vi "SkipIfLabVIEWVersionIsIncompatible.vi"(8 "error in (no error)":errorcluster, 10 "Minimum Version Year (2016)":string="2016", 11 "VeriStandTestCase in":refnum<class "VeriStandTestCase.lvclass">) -> (0 "error out":errorcluster, 2 "Skipped":bool, 3 "VeriStandTestCase out":refnum<class "VeriStandTestCase.lvclass">)   [LabVIEW 2027, in "VeriStandTestCase.lvclass"]
uses:
  VeriStandTestCase.lvclass
  <vilib>/addons/_JKI Toolkits/VI Tester/TestCase.llb/TestCase.lvclass
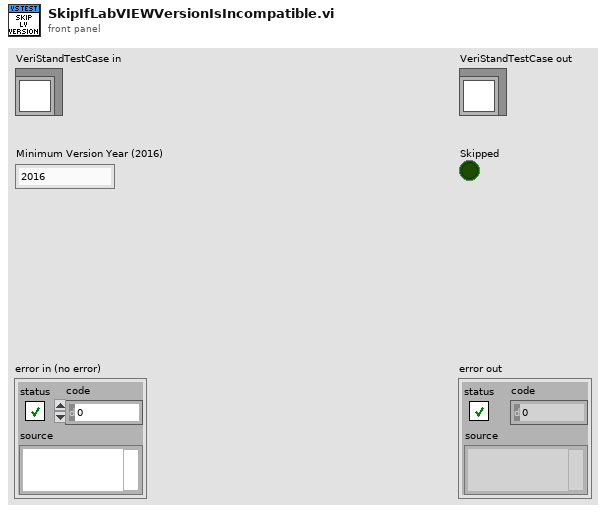
[diagram p1: front panel]
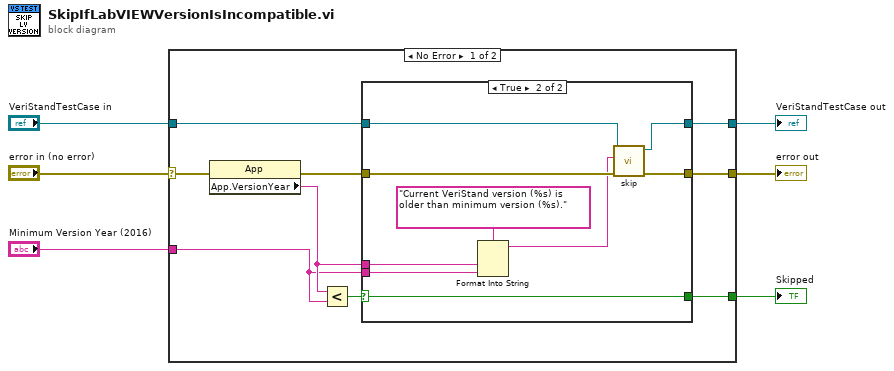
[diagram p0: block diagram]
diagram:
  n1 = case shown="No Error" "error in (no error)" {
    selector: "error in (no error)" -> [w11 w28]
    tunnel: [w9 w28] -> w5
    tunnel: [w12 w27] -> w3
    tunnel: "VeriStandTestCase in" -> [w13 w27]
    tunnel: "Minimum Version Year (2016)" -> [w8 _]
    tunnel: [w7 _] -> w1
    frame No Error {
      n2 = property class="App"(error in=w11) -> (error out=w10:errorcluster, "App.VersionYear"=w14:string)  [unwired: 1 in, 1 out]
      n3 = Less?(x=w14, y=w8) -> (x < y?=w15:bool)
      n4 = case shown="True" w15 {
        selector: w15 -> [_ w18]
        tunnel: w10 -> [w16 w26]
        tunnel: [w16 w25] -> w9
        tunnel: w13 -> [w17 w24]
        tunnel: [w17 w19] -> w12
        tunnel: w14 -> [_ w21]
        tunnel: w8 -> [_ w20]
        tunnel: [_ w18] -> w7
        frame False {
        }
        frame True {
          n5 = Format Into String(format string="Current VeriStand version (%s) is older than minimum version (%s).", w21, w20) -> (resulting string=w22:string)  [unwired: 2 in, 1 out]
          n6 = call <vilib>:"skip.vi"("error in (no error)"=w26, "skipMessage"=w22, "TestCase in"=w24) -> ("error out"=w25:errorcluster, "TestCase out"=w19:refnum<class "VeriStandTestCase.lvclass">)  [unwired: 7 in]
        }
      }
    }
    frame Error {
    }
  }
  "error out" <- w5
  "VeriStandTestCase out" <- w3
  "Skipped" <- w1
